vi "图片遍历显示.vi"() -> ()   [LabVIEW 2018]
panel:
  out "Resized Container":picture
  out "Resized Image":picture
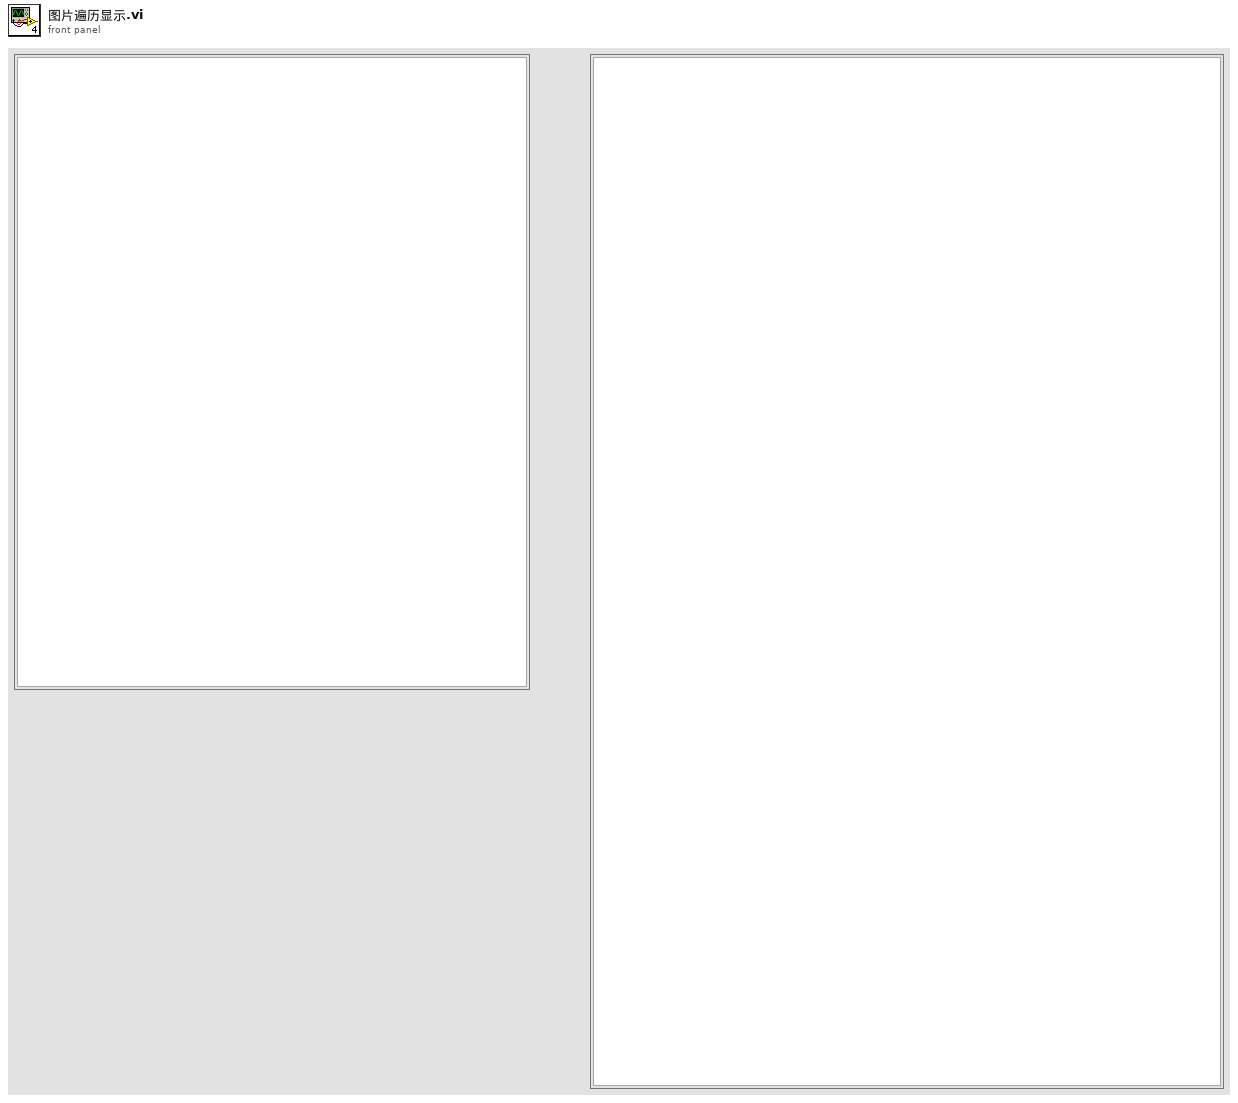
[diagram p1: front panel]
types:
  T1 = typedef "imagedata.ctl" = cluster{"image type":i32, "image depth":i32, "image":u8[], "mask":u8[], "colors":u32[], "Rectangle":cluster{"left":i16, "top":i16, "right":i16, "bottom":i16}}
  T2 = typedef "LVBoundsTypeDef.ctl" = cluster{"Width":u32, "Height":u32}
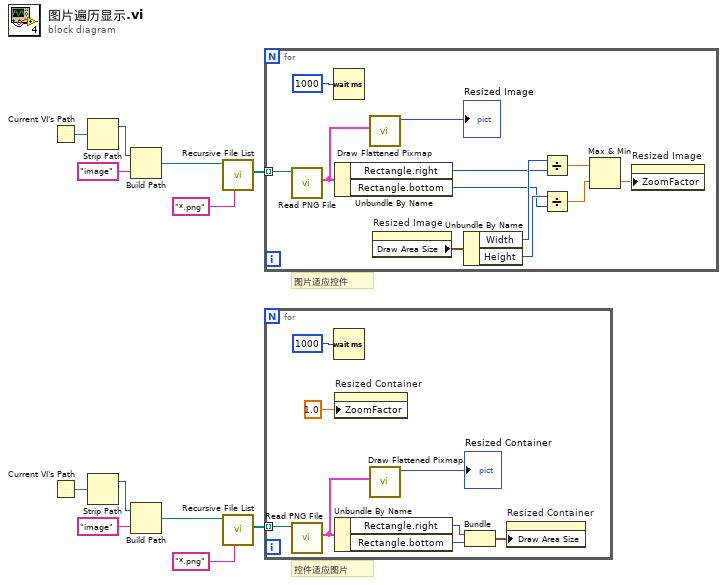
[diagram p0: block diagram]
diagram:
  # "控件适应图片"
  # "图片适应控件"
  n1 = Current VI's Path() -> (path=w12:path)
  n2 = Current VI's Path() -> (path=w1:path)
  n3 = Strip Path(path=w12) -> (stripped path=w11:path)  [unwired: 1 out]
  n4 = Strip Path(path=w1) -> (stripped path=w2:path)  [unwired: 1 out]
  n5 = Build Path(base path=w11, name or relative path="image" ("名称或相对路径")) -> (appended path=w9:path)
  n6 = Build Path(base path=w2, name or relative path="image" ("名称或相对路径")) -> (appended path=w4:path)
  n7 = call <vilib>:"Recursive File List.vi"("pattern"="*.png", "Folder Path"=w9) -> ("All Files in Dir"=w7:path[])  [unwired: 5 in, 4 out]
  n8 = call <vilib>:"Recursive File List.vi"("pattern"="*.png", "Folder Path"=w4) -> ("All Files in Dir"=w6:path[])  [unwired: 5 in, 4 out]
  n9 = for {
    tunnel: w7 -> [w24] mode=indexing
    n10 = call <vilib>:"Read PNG File.vi"("path to PNG file"=w24) -> ("image data"=w20:T1)  [unwired: 8 in, 2 out]
    n11 = Wait (ms)(milliseconds to wait=u32 1000 ("等待时间（毫秒）")) -> ()  [unwired: 1 out]
    n12 = Unbundle By Name(w20) -> ("Rectangle.right"=w18:i16, "Rectangle.bottom"=w16:i16)
    n13 = call <vilib>:"Draw Flattened Pixmap.vi"("image data"=w20) -> ("new picture"=→"Resized Image":picture)  [unwired: 8 in]
    n14 = property on="Resized Image" class="Pict"() -> ("Draw Area Size"=w21:T2)  [unwired: 2 in, 2 out]
    n15 = Unbundle By Name(w21) -> ("Width"=w19:u32, "Height"=w17:u32)
    n16 = Divide(x=w19, y=w18) -> (x/y=w15:dbl)
    n17 = Divide(x=w17, y=w16) -> (x/y=w14:dbl)
    n18 = Max & Min(x=w15, y=w14) -> (min(x,y)=w13:dbl)  [unwired: 1 out]
    n19 = property on="Resized Image" class="Pict"("ZoomFactor"=w13) -> ()  [unwired: 2 in, 2 out]
  }
  n20 = for {
    tunnel: w6 -> [w32] mode=indexing
    n21 = call <vilib>:"Read PNG File.vi"("path to PNG file"=w32) -> ("image data"=w29:T1)  [unwired: 8 in, 2 out]
    n22 = Wait (ms)(milliseconds to wait=u32 1000 ("等待时间（毫秒）")) -> ()  [unwired: 1 out]
    n23 = property on="Resized Container" class="Pict"("ZoomFactor"=sgl 1.0 ("缩放因子")) -> ()  [unwired: 2 in, 2 out]
    n24 = Unbundle By Name(w29) -> ("Rectangle.right"=w28:i16, "Rectangle.bottom"=w27:i16)
    n25 = call <vilib>:"Draw Flattened Pixmap.vi"("image data"=w29) -> ("new picture"=→"Resized Container":picture)  [unwired: 8 in]
    n26 = Bundle("right"=w28, "bottom"=w27) -> (w26:cluster{"right":i16, "bottom":i16})  [unwired: 1 in]
    n27 = property on="Resized Container" class="Pict"("Draw Area Size"=w26) -> ()  [unwired: 2 in, 2 out]
  }
